vi "CM51DriverServer.vi"   [LabVIEW 2010, in "CM51.lvlib"]
uses:
  CM51.lvlib
  Comunication Status.ctl
types:
  T1 = enum32{"Invalid", "Standard", "Closed", "Hidden", "Minimized", "Maximized"}
  T2 = typedef "CM51.lvlib/Comunication Status.ctl" = string
  T3 = typedef "CM51.lvlib/Serial Config.ctl" = cluster{"串口选择":refnum<visa-resource-name>, "通讯速率":u32, "超时时间":u32, "数据位长":u16, "奇偶校验":enum16{"None", "Odd", "Even", "Mark", "Space"}, "停止位长":u16, "握手控制":u16, "字符结束":bool, "结束字符":u8, "仪器地址":u32}
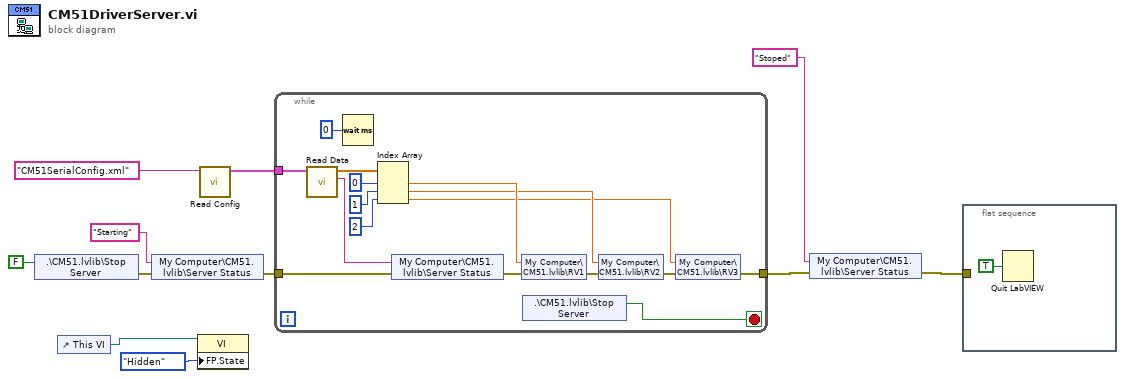
[diagram p0: block diagram]
diagram:
  n1 = shared-variable ".\\CM51.lvlib\\Stop Server"(FALSE ("Stop Server")) -> (error out=w7:errorcluster)  [unwired: 1 in]
  n2 = control-ref of="This VI"() -> (w2:refnum<vi>)
  n3 = shared-variable "My Computer\\CM51.lvlib\\Server Status"(T2 "Starting" ("Server Status"), error in=w7) -> (error out=w10:errorcluster)
  n4 = property class="VI"(reference=w2, "FP.State"=T1."Hidden" ("Front Panel Window:State")) -> ()  [unwired: 1 in, 2 out]
  n5 = call "Read Config.vi"("FileName"="CM51SerialConfig.xml") -> ("Serial Config"=w4:T3)  [unwired: 9 in, 1 out]
  n6 = while {
    tunnel: [w18] -> w11
    tunnel: w10 -> [w25]
    tunnel: w4 -> [w24]
    stop <- w26 stop-if-true
    n7 = call "Read Data.vi"("Serial Config"=w24) -> ("Status"=w22:string, "RV"=w23:dbl[])  [unwired: 8 in, 1 out]
    n8 = Wait (ms)(milliseconds to wait=u32 0) -> ()  [unwired: 1 out]
    n9 = Index Array(array=w23, index #1=0 ("index"), index #2=1 ("index"), index #3=2 ("index")) -> (element #1=w14:dbl, element #2=w13:dbl, element #3=w12:dbl)
    n10 = shared-variable "My Computer\\CM51.lvlib\\Server Status"(w22, error in=w25) -> (error out=w19:errorcluster)
    n11 = shared-variable "My Computer\\CM51.lvlib\\RV1"(w14, error in=w19) -> (error out=w21:errorcluster)
    n12 = shared-variable ".\\CM51.lvlib\\Stop Server"() -> (w26:bool)  [unwired: 1 in, 1 out]
    n13 = shared-variable "My Computer\\CM51.lvlib\\RV2"(w13, error in=w21) -> (error out=w20:errorcluster)
    n14 = shared-variable "My Computer\\CM51.lvlib\\RV3"(w12, error in=w20) -> (error out=w18:errorcluster)
  }
  n15 = shared-variable "My Computer\\CM51.lvlib\\Server Status"(T2 "Stoped" ("Server Status"), error in=w11) -> (error out=w3:errorcluster)
  n16 = flat-sequence {
    tunnel: w3 -> [_]
    frame #0 {
      n17 = Quit LabVIEW(quit? (T)=TRUE) -> ()
    }
  }
